vi "Configure Serial Output Reference Clock Frequency.vi"(0 "fpga interface in":refnum<k20>, 5 "serial output channels":string[](array[string]), 7 "serial output reference clock frequency (Hz)":dbl=25000000.0 format="%#_6p", 11 "error in (no error)":errorcluster) -> (4 "fpga interface out":refnum<k20>, 15 "error out":errorcluster)   [LabVIEW 2023, in "GettingStarted_Common_148X_Host.lvlib"]
uses:
  GettingStarted_Common_148X_Host.lvlib
  5b561469-cbe9-467f-a4ba-3c9d6b12c712.vi
  <instrlib>/FlexRIO/API/Host/v1/NI FlexRIO/API/Get Property Reference - Fpga Small.vi
  <resource>/objmgr/niflexrioapiChannel.rc
  <instrlib>/FlexRIO/API/Host/v1/NI FlexRIO API v1.lvlib
  <resource>/objmgr/niflexrioapiClock.rc
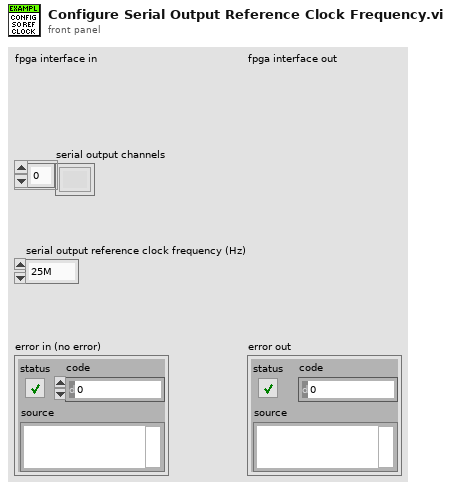
[diagram p1: front panel]
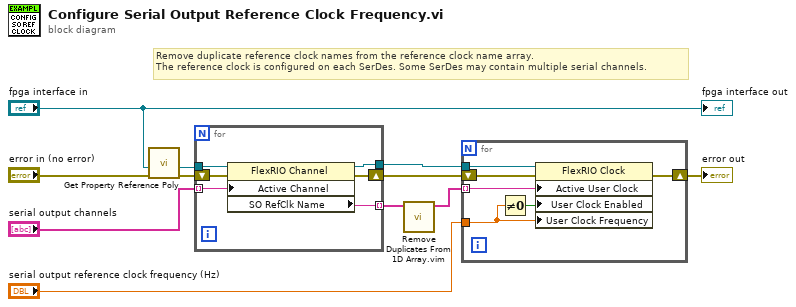
[diagram p0: block diagram]
diagram:
  # "Remove duplicate reference clock names from the reference clock name array.\nThe reference clock is configured on each SerDes. Some SerDes may contain multiple serial channels."
  n1 = call-poly <instrlib>:"Get Property Reference Poly.vi"("error in (no error)"="error in (no error)", "fpga interface in"="fpga interface in") -> ("error out"=w5:errorcluster, "property reference"=w6:refnum<k20>)  [unwired: 4 in, 1 out]
  n2 = for {
    tunnel: "serial output channels" -> [w12] mode=indexing
    tunnel: [w13] -> w3 mode=indexing
    shift-right: [w16] -> w10
    shift-left: w5 -> [w14]
    tunnel: w6 -> [w15]
    tunnel: [w17] -> w11
    n3 = property class="FlexRIO Channel"(reference=w15, error in=w14, "Active Channel"=w12) -> (reference out=w17:refnum<k20>, error out=w16:errorcluster, "SO RefClk Name"=w13:string)
  }
  n4 = call "Remove Duplicates From 1D Array.vim"("array"=w3) -> ("array with duplicates removed"=w2:string[])  [unwired: 10 in]
  n5 = for {
    tunnel: w11 -> [w23]
    shift-right: [w21] -> w8
    shift-left: w10 -> [w22]
    tunnel: w2 -> [w19] mode=indexing
    tunnel: "serial output reference clock frequency (Hz)" -> [w18]
    n6 = Not Equal To 0?(x=w18) -> (x != 0?=w20:bool)
    n7 = property class="FlexRIO Clock"(reference=w23, error in=w22, "Active User Clock"=w19, "User Clock Enabled"=w20, "User Clock Frequency"=w18) -> (error out=w21:errorcluster)  [unwired: 1 out]
  }
  "error out" <- w8
  "fpga interface out" <- "fpga interface in"
